vi "executeStrategy.vi"(8 "error in (no error)":errorcluster, 9 "num2":dbl, 10 "num1":dbl, 11 "Context in":refnum<class "Context.lvclass">) -> (0 "error out":errorcluster, 3 "Context out":refnum<class "Context.lvclass">)   [LabVIEW 2018, in "Context.lvclass"]
uses:
  Context.lvclass
  Context.lvclass/Context.ctl
  Strategy Class/Strategy.lvclass
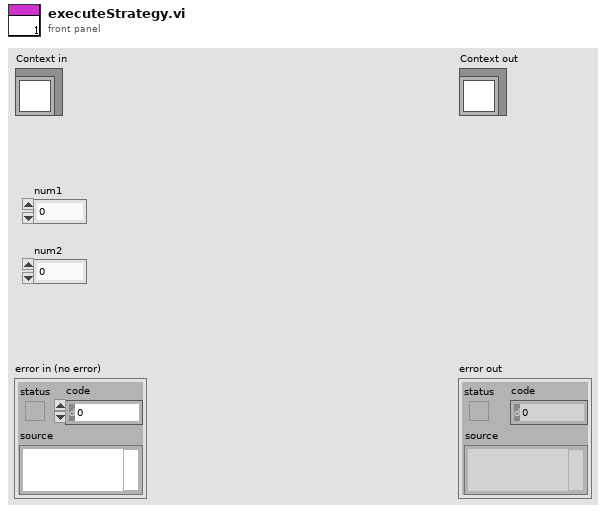
[diagram p1: front panel]
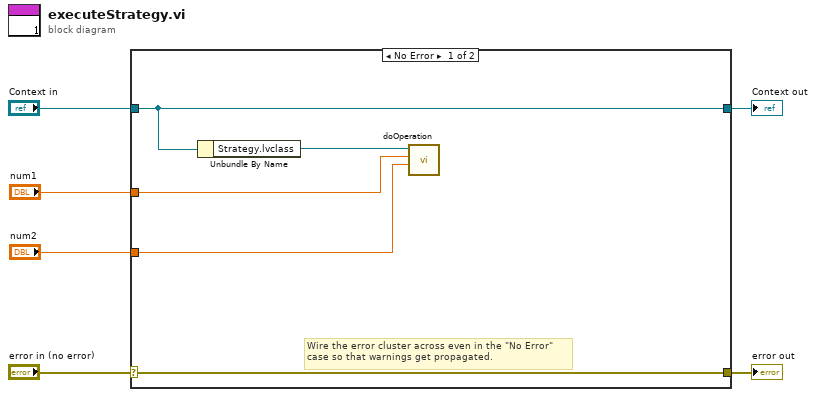
[diagram p0: block diagram]
diagram:
  n1 = case shown="No Error" "error in (no error)" {
    selector: "error in (no error)" -> [w11 w13]
    tunnel: [w11 w13] -> w5
    tunnel: [w10 w12] -> w3
    tunnel: "Context in" -> [w10 w12]
    tunnel: "num1" -> [w8 _]
    tunnel: "num2" -> [w7 _]
    frame No Error {
      # "Wire the error cluster across even in the \"No Error\"\ncase so that warnings get propagated."
      n2 = Unbundle By Name(w10) -> ("Strategy.lvclass"=w9:refnum<class "Strategy.lvclass">)
      n3 = call-dynamic "doOperation.vi"("num2"=w7, "num1"=w8, "Strategy in"=w9) -> ()  [unwired: 7 in, 2 out]
    }
    frame Error {
    }
  }
  "error out" <- w5
  "Context out" <- w3
